vi "Update Scalar Channel Properties.vi"(8 "error in (no error)":errorcluster, 9 "new bitfile scalar channel":T4 {"Data Type" format="%.0x"}, 10 "old bitfile scalar channel":T1 {"Item Ref" format="%.0x"}) -> (0 "error out":errorcluster, 2 "scalar channel out":T1 {"Item Ref" format="%.0x"}, 5 "remove":bool)   [LabVIEW 2018, in "FPGA Addon System Explorer.lvlib"]
uses:
  FPGA Addon System Explorer.lvlib
  Addon Shared/Types/Register Information.ctl
  Addon Shared/Types/Data Type.ctl
  Types/Output Scalar.ctl
  <vilib>/NI Veristand/Custom Device API/Custom Device Item Ref.ctl
  <vilib>/NI Veristand/Custom Device API/Custom Device API.lvlib
  Addon Shared/FPGA Addon Shared.lvlib
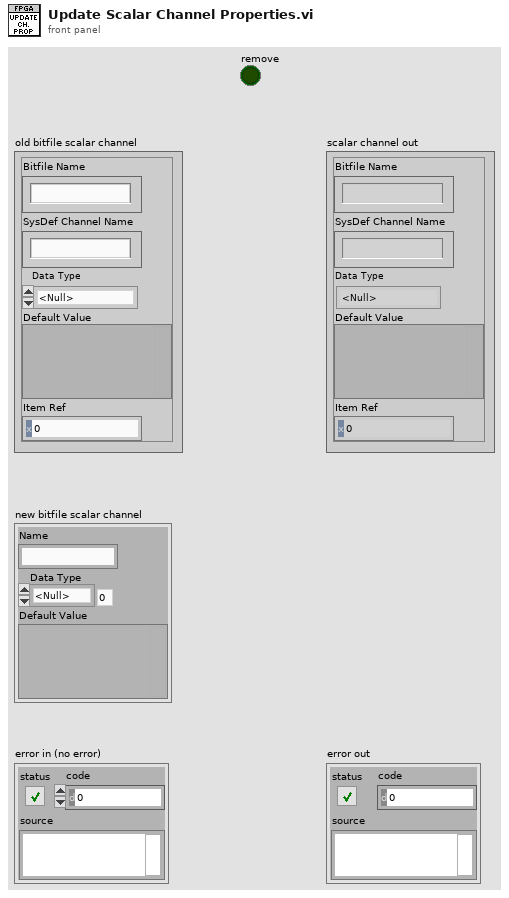
[diagram p1: front panel]
types:
  T1 = typedef "FPGA Addon System Explorer.lvlib/Output Scalar.ctl" = cluster{"Bitfile Name":string, "SysDef Channel Name":string, "Data Type":T2, "Default Value":variant, "Item Ref":T3}
  T2 = typedef "FPGA Addon Shared.lvlib/Data Type.ctl" = enum8{"<Null>", "I8", "I16", "I32", "I64", "U8", "U16", "U32", "U64", "SGL", "Boolean", "Analog PWM In Settings", "Analog PWM In", "Digital PWM In Settings", "Digital PWM In", "Digital PWM Out", "Sine Out", "FXP+/-24.5", "FXP+/-16.5", "FXP+/-32.8", "FXP+/-64.32", "FXP+/-16.7", "FXP+/-20.5", "FXP+/-27.5", "FXP+/-32.16", "FXP+16.3", "FXP+18.3", "Digital Static In", "Digital Static Out", "Digital Static In Settings", "Digital WSS Out", "Quad Encoder Settings", "Quad Encoder In", "Group"}
  T3 = typedef "Custom Device API.lvlib/Custom Device Item Ref.ctl" = u64
  T4 = typedef "FPGA Addon Shared.lvlib/Register Information.ctl" = cluster{"Name":string, "Data Type":T2, "Default Value":variant}
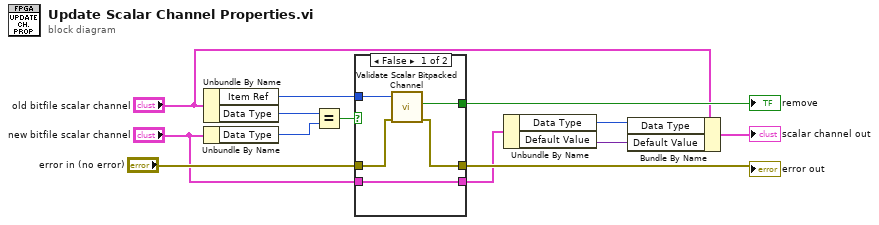
[diagram p0: block diagram]
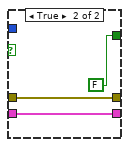
[diagram p2: hidden frame]
diagram:
  n1 = Unbundle By Name("old bitfile scalar channel") -> ("Item Ref"=w9:T3, "Data Type"=w13:T2)
  n2 = Unbundle By Name("new bitfile scalar channel") -> ("Data Type"=w10:T2)
  n3 = Equal?(x=w13, y=w10) -> (x = y?=w11:bool)
  n4 = case shown="False" w11 {
    tunnel: "error in (no error)" -> [w17 w21]
    tunnel: w9 -> [w18 _]
    tunnel: [w16 w21] -> w8
    tunnel: [w15 FALSE ("bitpacked")] -> w7
    tunnel: "new bitfile scalar channel" -> [w14 w19]
    tunnel: [w14 w19] -> w5
    frame False {
      n5 = call "Validate Scalar Bitpacked Channel.vi"("error in (no error)"=w17, "Item Ref"=w18) -> ("error out"=w16:errorcluster, "bitpacked"=w15:bool)  [unwired: 7 in, 1 out]
    }
    frame True {
    }
  }
  "error out" <- w8
  "remove" <- w7
  n6 = Unbundle By Name(w5) -> ("Data Type"=w2:T2, "Default Value"=w3:variant)
  n7 = Bundle By Name(cluster="old bitfile scalar channel", "Data Type"=w2, "Default Value"=w3) -> (→"scalar channel out":T1)
